vi "Init Project VIs List.vi"(4 "unmark button":refnum<vi>, 5 "mark button":refnum<vi>, 6 "String Unmarked":string, 7 "String Marked":string, 8 "error in":errorcluster, 10 "Project Contents":T1, 11 "list in":refnum<vi>) -> (0 "error out":errorcluster, 3 "list out":refnum<vi>)   [LabVIEW 2020]
uses:
  <vilib>/SourceOnly/NI_SourceOnly_CollectionOfVIsAndLibraries.ctl
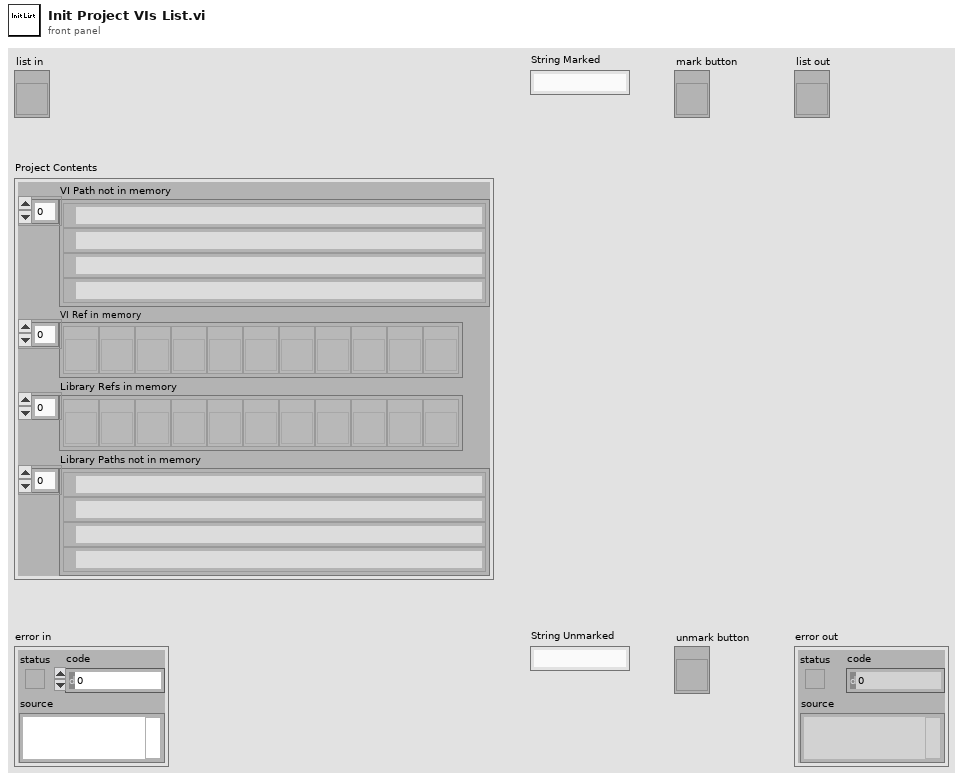
[diagram p1: front panel]
types:
  T1 = typedef "NI_SourceOnly_CollectionOfVIsAndLibraries.ctl" = cluster{"VI Path not in memory":path[], "VI Ref in memory":refnum<vi>[], "Library Refs in memory":refnum<vi>[], "Library Paths not in memory":path[]}
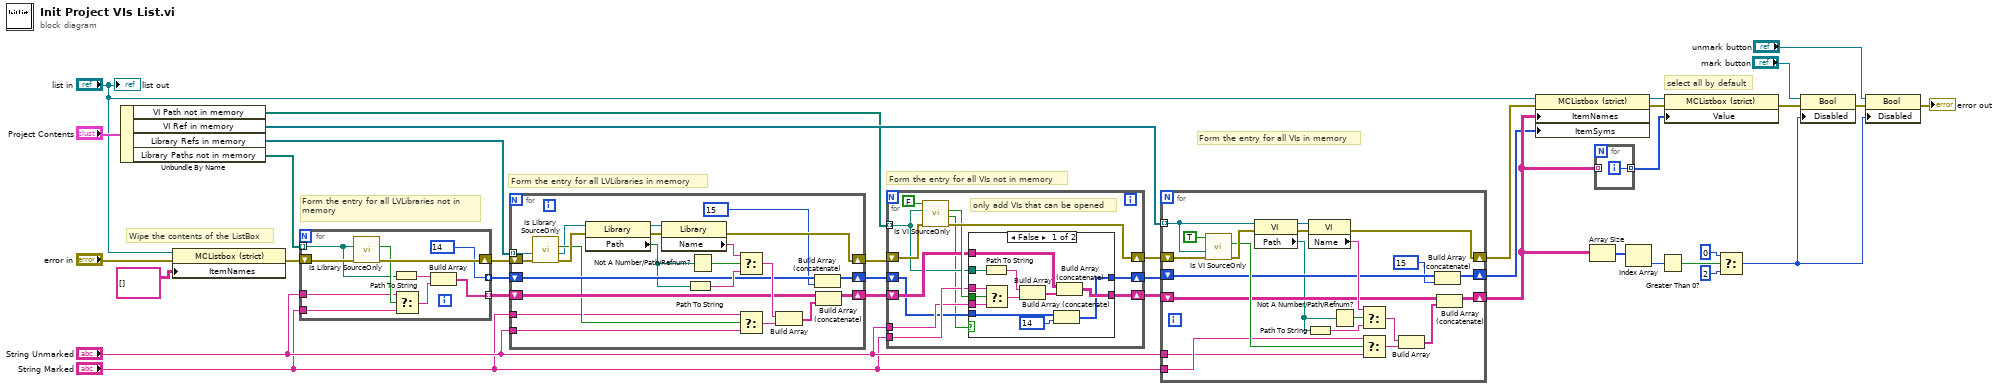
[diagram p0: block diagram]
diagram:
  # "Form the entry for all VIs in memory"
  # "Form the entry for all VIs not in memory"
  # "Form the entry for all LVLibraries in memory"
  # "Form the entry for all LVLibraries not in memory"
  # "Wipe the contents of the ListBox"
  # "select all by default"
  n1 = Unbundle By Name("Project Contents") -> ("VI Path not in memory"=w23:path[], "VI Ref in memory"=w26:refnum<vi>[], "Library Refs in memory"=w9:refnum<vi>[], "Library Paths not in memory"=w6:path[])
  n2 = property class="MCListbox (strict)"(reference="list in", error in="error in", "ItemNames"=string[][] [] ("Item Names")) -> (error out=w28:errorcluster)  [unwired: 1 out]
  n3 = for {
    shift-right: [w46] -> w29
    shift-left: w28 -> [w47]
    tunnel: "String Unmarked" -> [w43]
    tunnel: "String Marked" -> [w42]
    tunnel: w6 -> [w41] mode=indexing
    tunnel: [14] -> w2 mode=indexing
    tunnel: [w38] -> w1 mode=indexing
    n4 = call <vilib>:"Is Library SourceOnly.vi"("error in"=w47, "Library Path"=w41) -> ("error out"=w46:errorcluster, "Is SourceOnly?"=w44:bool)  [unwired: 7 in, 1 out]
    n5 = Path To String(path=w41) -> (string=w40:string)
    n6 = Select(t=w43, s=w44, f=w42) -> (s? t:f=w45:string)
    n7 = Build Array(w40, w45) -> (w38:string[])
  }
  n8 = for {
    shift-right: [w68] -> w30
    shift-left: w29 -> [w67]
    shift-right: [w56] -> w10
    shift-left: w1 -> [w58]
    shift-right: [w55] -> w11
    shift-left: w2 -> [w57]
    tunnel: w9 -> [w53] mode=indexing
    tunnel: "String Marked" -> [w51]
    tunnel: "String Unmarked" -> [w50]
    n9 = call <vilib>:"Is Library SourceOnly.vi"("error in"=w67, "Library Ref in"=w53) -> ("error out"=w66:errorcluster, "Library Ref out"=w52:refnum<vi>, "Is SourceOnly?"=w54:bool)  [unwired: 7 in]
    n10 = property class="Library"(reference=w52, error in=w66) -> (reference out=w64:refnum<vi>, error out=w69:errorcluster, "Path"=w48:path)
    n11 = property class="Library"(reference=w64, error in=w69) -> (error out=w68:errorcluster, "Name"=w63:string)  [unwired: 1 out]
    n12 = Path To String(path=w48) -> (string=w62:string)
    n13 = Not A Number/Path/Refnum?(number/path/refnum=w48) -> (NaN/Path/Refnum?=w65:bool)
    n14 = Select(t=w63, s=w65, f=w62) -> (s? t:f=w61:string)
    n15 = Select(t=w51, s=w54, f=w50) -> (s? t:f=w59:string)
    n16 = Build Array(w61, w59) -> (w60:string[])
    n17 = Build Array (concatenate)(w57, 15) -> (w55:i32[])
    n18 = Build Array (concatenate)(w58, w60) -> (w56:string[][])
  }
  n19 = for {
    tunnel: w23 -> [w71] mode=indexing
    shift-right: [w80] -> w35
    shift-left: w30 -> [w81]
    tunnel: "String Marked" -> [w77]
    tunnel: "String Unmarked" -> [w76]
    shift-right: [w73] -> w25
    shift-left: w10 -> [w75]
    shift-right: [w72] -> w24
    shift-left: w11 -> [w74]
    # "only add VIs that can be opened"
    n20 = call <vilib>:"Is VI SourceOnly.vi"("error in (no error)"=w81, "VI Path"=w71, "Is VI in Memory"=FALSE) -> ("error out"=w80:errorcluster, "Version Error"=w70:bool, "Is SourceOnly?"=w78:bool)  [unwired: 1 in, 5 out]
    n21 = case shown="False" w70 {
      tunnel: w78 -> [w91 _]
      tunnel: w77 -> [w90 _]
      tunnel: w76 -> [w89 _]
      tunnel: w75 -> [w87 w94]
      tunnel: w74 -> [w86 w95]
      tunnel: [w85 w94] -> w73
      tunnel: [w84 w95] -> w72
      tunnel: w71 -> [w82 _]
      frame False {
        n22 = Path To String(path=w82) -> (string=w93:string)
        n23 = Select(t=w90, s=w91, f=w89) -> (s? t:f=w88:string)
        n24 = Build Array(w93, w88) -> (w92:string[])
        n25 = Build Array (concatenate)(w86, 14) -> (w84:i32[])
        n26 = Build Array (concatenate)(w87, w92) -> (w85:string[][])
      }
      frame True {
      }
    }
  }
  n27 = for {
    tunnel: w26 -> [w107] mode=indexing
    shift-right: [w114] -> w31
    shift-left: w35 -> [w116]
    tunnel: "String Marked" -> [w104]
    tunnel: "String Unmarked" -> [w103]
    shift-right: [w99] -> w13
    shift-left: w25 -> [w101]
    shift-right: [w98] -> w12
    shift-left: w24 -> [w100]
    n28 = call <vilib>:"Is VI SourceOnly.vi"("error in (no error)"=w116, "VI ref"=w107, "Is VI in Memory"=TRUE) -> ("error out"=w115:errorcluster, "Is SourceOnly?"=w105:bool)  [unwired: 1 in, 6 out]
    n29 = property class="VI"(reference=w107, error in=w115) -> (reference out=w112:refnum<vi>, error out=w117:errorcluster, "Path"=w96:path)
    n30 = Path To String(path=w96) -> (string=w110:string)
    n31 = property class="VI"(reference=w112, error in=w117) -> (error out=w114:errorcluster, "Name"=w111:string)  [unwired: 1 out]
    n32 = Not A Number/Path/Refnum?(number/path/refnum=w96) -> (NaN/Path/Refnum?=w113:bool)
    n33 = Select(t=w111, s=w113, f=w110) -> (s? t:f=w109:string)
    n34 = Select(t=w104, s=w105, f=w103) -> (s? t:f=w102:string)
    n35 = Build Array(w109, w102) -> (w108:string[])
    n36 = Build Array (concatenate)(w100, 15) -> (w98:i32[])
    n37 = Build Array (concatenate)(w101, w108) -> (w99:string[][])
  }
  n38 = property class="MCListbox (strict)"(reference="list in", error in=w31, "ItemNames"=w13, "ItemSyms"=w12) -> (reference out=w22:refnum<vi>, error out=w34:errorcluster)
  n39 = Array Size(array=w13) -> (size(s)=w20:i32[])
  n40 = for {
    tunnel: w13 -> [_] mode=indexing
    tunnel: [w118] -> w5 mode=indexing
    i -> [w118]
  }
  n41 = Index Array(array=w20) -> (element=w19:i32)  [unwired: 1 in]
  n42 = Greater Than 0?(x=w19) -> (x > 0?=w18:bool)
  n43 = property class="MCListbox (strict)"(reference=w22, error in=w34, "Value"=w5) -> (error out=w32:errorcluster)  [unwired: 1 out]
  n44 = Select(t=u8 0 ("Disabled"), s=w18, f=u8 2) -> (s? t:f=w14:u8)
  n45 = property class="Bool"(reference="mark button", error in=w32, "Disabled"=w14) -> (error out=w33:errorcluster)  [unwired: 1 out]
  n46 = property class="Bool"(reference="unmark button", error in=w33, "Disabled"=w14) -> (error out=→"error out":errorcluster)  [unwired: 1 out]
  "list out" <- "list in"
